vi "sec_Log_main.vi"(7 "Command":T2, 8 "error in (no error)":errorcluster, 10 "Alarm States":T1[](array[typedef]), 11 "Number Of Alarms":i32) -> (0 "error out":errorcluster)   [LabVIEW 2009]
doc: "This Module is responsible for updating the Alarm Log when an Alarm has changed State\nThe file appears in the ..\\data folder relative to the application directory\nFile name is \"alarm.log.txt\"\nDate, Time, Zone and Status are logging to disk"
uses:
  sec_Log_Command_enum.ctl
  controls/sec_AlarmStates_enum.ctl
panel:
  # "Inputs"
  # "Outputs"
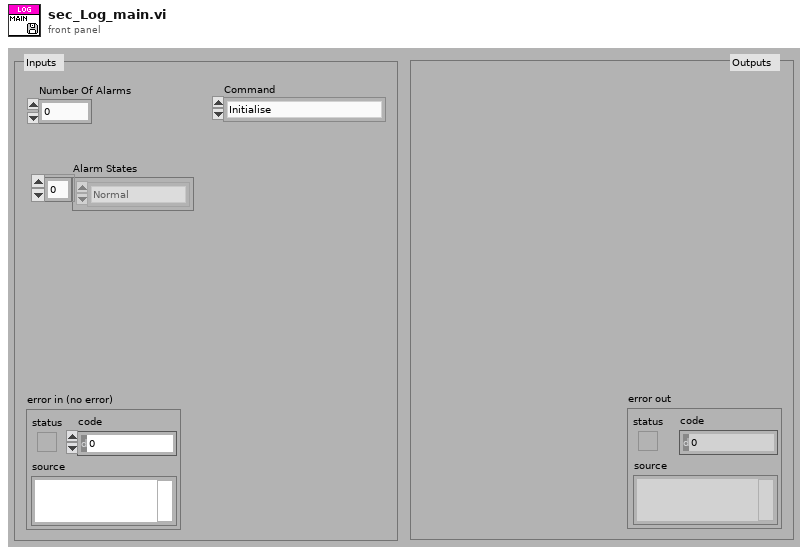
[diagram p1: front panel]
types:
  T1 = typedef "sec_AlarmStates_enum.ctl" = enum16{"Normal", "Alarm", "Bypass", "Tamper"}
  T2 = typedef "sec_Log_Command_enum.ctl" = enum16{"Initialise", "Log Alarms"}
  T3 = enum16{"open", "replace", "create", "open or create", "replace or create", "replace or create with confirmation"}
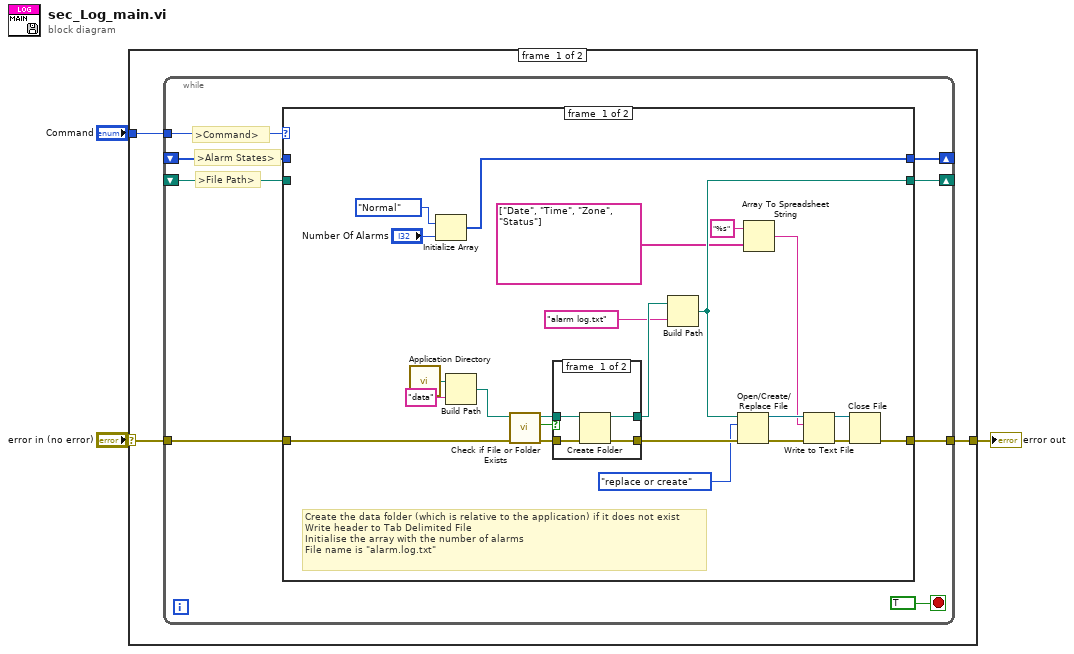
[diagram p0: block diagram]
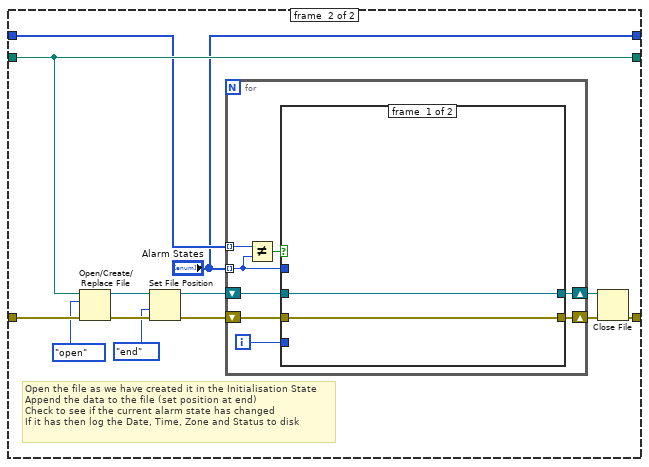
[diagram p3: hidden frame]
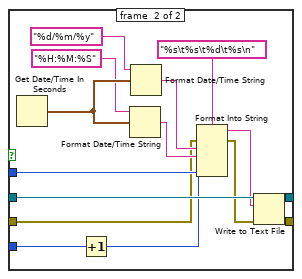
[diagram p4: hidden frame]
diagram:
  n1 = case shown="No Error" "error in (no error)" {
    selector: "error in (no error)" -> [w5 w82]
    tunnel: [w6 w82] -> w2
    tunnel: "Command" -> [w4 _]
    frame #0 {
      n2 = while {
        tunnel: [w14] -> w6
        tunnel: w5 -> [w13]
        tunnel: w4 -> [w12]
        shift-right: [w11] -> _
        shift-left: _ -> [w10]
        shift-right: [w8] -> _
        shift-left: _ -> [w7]
        stop <- TRUE stop-if-true
        # ">File Path>"
        # ">Alarm States>"
        # ">Command>"
        n3 = case shown="\"Initialise\", Default" w12 {
          tunnel: [w28 w51] -> w14
          tunnel: w13 -> [w34 w55]
          tunnel: [w15 "Alarm States"] -> w11
          tunnel: w10 -> [_ w50]
          tunnel: [w21 w56] -> w8
          tunnel: w7 -> [_ w56]
          frame #0 {
            # "Create the data folder (which is relative to the application) if it does not exist\nWrite header to Tab Delimited File\nInitialise the array with the number of alarms\nFile name is \"alarm.log.txt\""
            n4 = call <vilib>:"Application Directory.vi"() -> ("Application Directory"=w37:path)
            n5 = Initialize Array(sec_AlarmStates_enum."Normal" ("Alarm State"), "Number Of Alarms") -> (w15:T1[])
            n6 = Build Path(base path=w37, name or relative path="data") -> (appended path=w35:path)
            n7 = call <vilib>:"Check if File or Folder Exists.vi"("error in (no error)"=w34, "path"=w35) -> ("error out"=w32:errorcluster, "file or folder exists?"=w33:bool, "dup path"=w31:path)  [unwired: 7 in]
            n8 = case shown="False" w33 {
              tunnel: w32 -> [w41 w43]
              tunnel: [w40 w43] -> w27
              tunnel: w31 -> [w39 w42]
              tunnel: [w38 w42] -> w24
              frame #0 {
                n9 = Create Folder(path (use dialog)=w39, error in=w41) -> (created path=w38:path, error out=w40:errorcluster)  [unwired: 1 in, 1 out]
              }
              frame #1 {
              }
            }
            n10 = Build Path(base path=w24, name or relative path="alarm log.txt") -> (appended path=w21:path)
            n11 = Open/Create/Replace File(file path (use dialog)=w21, error in=w27, operation (0:open)=T3."replace or create") -> (refnum out=w26:refnum<file>, error out=w30:errorcluster)  [unwired: 3 in, 1 out]
            n12 = Array To Spreadsheet String(array=string[] ["Date", "Time", "Zone", "Status"], 3:"%s" ("format string")) -> (spreadsheet string=w18:string)  [unwired: 1 in]
            n13 = Write to Text File(file (use dialog)=w26, text=w18, error in=w30) -> (refnum out=w25:refnum<file>, error out=w29:errorcluster)  [unwired: 1 in, 1 out]
            n14 = Close File(refnum=w25, error in=w29) -> (error out=w28:errorcluster)  [unwired: 1 out]
          }
          frame #1 {
            # "Open the file as we have created it in the Initialisation State\nAppend the data to the file (set position at end)\nCheck to see if the current alarm state has changed\nIf it has then log the Date, Time, Zone and Status to disk"
            n15 = Open/Create/Replace File(file path (use dialog)=w56, error in=w55, operation (0:open)=T3."open") -> (refnum out=w48:refnum<file>, error out=w46:errorcluster)  [unwired: 3 in, 1 out]
            n16 = Set File Position(refnum=w48, from (0:start)=enum16{"start", "end", "current"}."end", error in=w46) -> (refnum out=w47:refnum<file>, error out=w45:errorcluster)  [unwired: 1 in]
            n17 = for {
              shift-right: [w62] -> w52
              shift-left: w45 -> [w63]
              shift-right: [w61] -> w53
              shift-left: w47 -> [w64]
              tunnel: "Alarm States" -> [w58] mode=indexing
              tunnel: w50 -> [w60] mode=indexing
              i -> [w57]
              n18 = Not Equal?(x=w60, y=w58) -> (x != y?=w59:bool)
              n19 = case shown="True" w59 {
                tunnel: w64 -> [w65 w81]
                tunnel: w63 -> [w66 w69]
                tunnel: [w66 w80] -> w62
                tunnel: [w65 w79] -> w61
                tunnel: w58 -> [_ w75]
                tunnel: w57 -> [_ w74]
                frame #0 {
                }
                frame #1 {
                  n20 = Get Date/Time In Seconds() -> (seconds since 1Jan1904=w77:timestamp)
                  n21 = Increment(x=w74) -> (x+1=w67:i32)
                  n22 = Format Date/Time String(time format string (%c)="%H:%M:%S", seconds (now)=w77) -> (date/time string=w73:string)  [unwired: 1 in]
                  n23 = Format Date/Time String(time format string (%c)="%d/%m/%y", seconds (now)=w77) -> (date/time string=w72:string)  [unwired: 1 in]
                  n24 = Format Into String(format string="%s\t%s\t%d\t%s\n", error in=w69, w72, w73, w67, w75) -> (resulting string=w70:string, error out=w68:errorcluster)  [unwired: 1 in]
                  n25 = Write to Text File(file (use dialog)=w81, text=w70, error in=w68) -> (refnum out=w79:refnum<file>, error out=w80:errorcluster)  [unwired: 1 in, 1 out]
                }
              }
            }
            n26 = Close File(refnum=w53, error in=w52) -> (error out=w51:errorcluster)  [unwired: 1 out]
          }
        }
      }
    }
    frame #1 {
    }
  }
  "error out" <- w2
